vi "Unflatten.vi"(8 "error in (no error)":errorcluster, 9 "timeout in":bool, 11 "CIFfifo in":refnum<class "CIFfifo.lvclass">) -> (0 "error out":errorcluster, 1 "Header":T1, 2 "Data":u8[](array[numeric]) format="%.0x", 3 "CIFfifo out":refnum<class "CIFfifo.lvclass">)   [LabVIEW 2021, in "CIFfifo.lvclass"]
uses:
  CIFfifo.lvclass
  typedef/FIFO Header.ctl
  CIFfifo.lvclass/CIFfifo.ctl
  Accessors/Write Header.vi
  <vilib>/CIF Foundation/CIF Utilities/DataTypes/Unflatten U64.vi
  <vilib>/CIF Foundation/CIF Utilities/DataTypes/Unflatten I64.vi
  ChannelCommon.lvlib
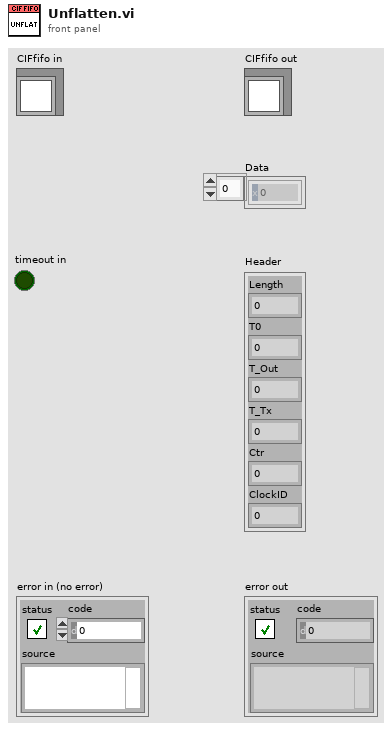
[diagram p1: front panel]
types:
  T1 = typedef "ChannelCommon.lvlib/FIFO Header.ctl" = cluster{"Length":u64, "T0":i64, "T_Out":i64, "T_Tx":i64, "Ctr":u64, "ClockID":u8}
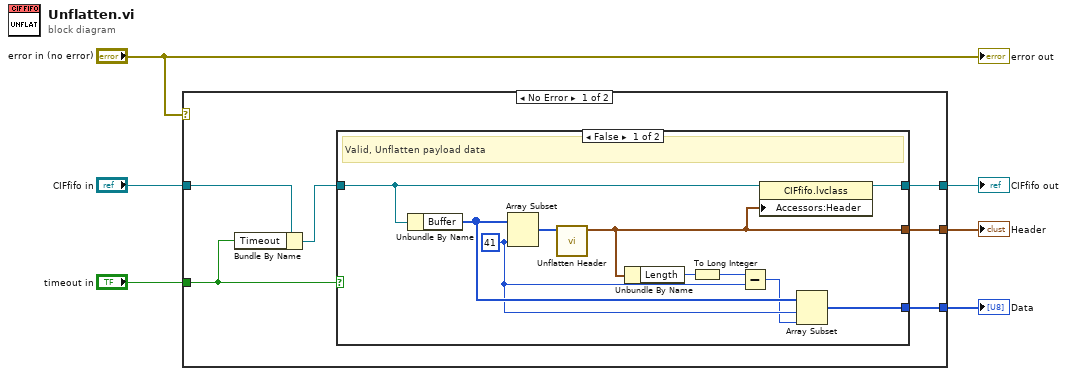
[diagram p0: block diagram]
diagram:
  n1 = case shown="No Error" "error in (no error)" {
    tunnel: [w8 w24] -> w2
    tunnel: "CIFfifo in" -> [w12 w24]
    tunnel: "timeout in" -> [w7 _]
    tunnel: [w10 _] -> w4
    tunnel: [w9 _] -> w5
    frame No Error {
      n2 = Bundle By Name(cluster=w12, "Timeout"=w7) -> (w11:refnum<class "CIFfifo.lvclass">)
      n3 = case shown="False" w7 {
        tunnel: w11 -> [w22 w23]
        tunnel: [w17 _] -> w10
        tunnel: [w18 _] -> w9
        tunnel: [w21 w23] -> w8
        frame False {
          w15 = 41 ("index")
          # "Valid, Unflatten payload data"
          n4 = Unbundle By Name(w22) -> ("Buffer"=w19:u8[])
          n5 = Array Subset(array=w19, length=w15) -> (w20:u8[])  [unwired: 1 in]
          n6 = call "Unflatten Header.vi"("Flattened Data in"=w20) -> ("Header out"=w18:T1)  [unwired: 9 in, 1 out]
          n7 = Unbundle By Name(w18) -> ("Length"=w16:u64)
          n8 = To Long Integer(number=w16) -> (32bit integer=w13:i32)
          n9 = Subtract(x=w13, y=w15) -> (x-y=w14:i32)
          n10 = property class="CIFfifo.lvclass"(reference=w22, "Accessors:Header"=w18) -> (reference out=w21:refnum<class "CIFfifo.lvclass">)  [unwired: 1 in, 1 out]
          n11 = Array Subset(array=w19, index=w15, length=w14) -> (w17:u8[])
        }
        frame True {
          # "Timeout"
        }
      }
    }
    frame Error {
    }
  }
  "CIFfifo out" <- w2
  "Header" <- w5
  "Data" <- w4
  "error out" <- "error in (no error)"
